vi "SoftwareBreakpoint.vi"(0 "Motion Board ID":T2=1 min=1 max=32 step=1, 1 "Axis or Vector Space":T1=1 items=["Axis 1"=1, "Axis 2"=2, "Axis 3"=3, "Axis 4"=4, "Axis 5"=5, "Axis 6"=6, "Axis 7"=7, "Axis 8"=8, "Vector Space 1"=17, "Vector Space 2"=18, "Vector Space 3"=19, "Vector Space 4"=20], 2 "Start Position":i32=500, 3 "Breakpoint Modulus":i32=500, 4 "error in (no error)":errorcluster) -> (6 "Breakpoints Occured":i32)   [LabVIEW 2022 SP3]
uses:
  <vilib>/Motion/FlexMotion/CustomControls/CustomControls.llb/AxisOrVectorSpace To Control.flx
panel:
  out "BreakPT marks":i32[](array[numeric])
  out "Current Position":i32=2000
  # "Enter a breakpoint Modulus, and the\nBreakpoint Output will occur at 0 and\nincrements of the Modulus Value."
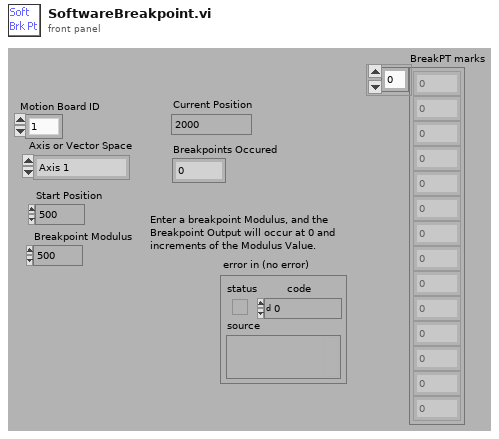
[diagram p1: front panel]
types:
  T1 = typedef "AxisOrVectorSpace To Control.flx" = u16
  T2 = typedef "Board Id" = u8
  T3 = typedef "Resource Out (Enum).flx" = u16
  T4 = typedef "Bd Id Out" = u8
  T5 = cluster{"Run/Stop":bool, "Profile Complete":bool, "Motor Off ":bool, "Following Error":bool, "Limit Switch":bool, "Home Switch":bool, "SW Limit Switch":bool, "Watchdog":bool, "Velocity Threshold":bool, "Position Brkpt":bool, "Home Found":bool, "Index Found":bool, "High Speed Capture":bool, "Reverse Direction":bool, "Blend Complete":bool, "Move Complete":bool}
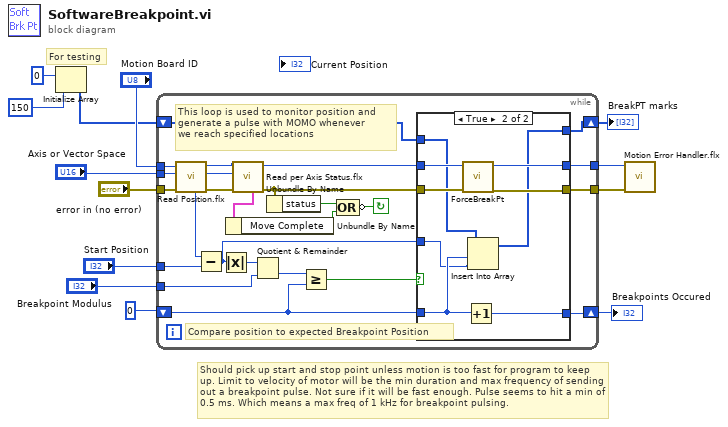
[diagram p0: block diagram]
diagram:
  # "For testing"
  # "Should pick up start and stop point unless motion is too fast for program to keep up. Limit to velocity of motor will be the min duration and max frequency of sending out a breakpoint pulse. Not sure if it will be fast enough. Pulse seems to hit a min of 0.5 ms. Which means a max freq of 1 kHz for breakpoint pulsing."
  n1 = Initialize Array(0, 150) -> (w2:i32[])
  n2 = while {
    shift-left: 0 -> [w18]
    shift-right: [w23] -> w7
    tunnel: "Axis or Vector Space" -> [w26]
    tunnel: "Motion Board ID" -> [w27]
    tunnel: [w28] -> w10
    tunnel: [w29] -> w11
    tunnel: "error in (no error)" -> [w24]
    tunnel: "Breakpoint Modulus" -> [w21]
    tunnel: "Start Position" -> [w20]
    shift-right: [w14] -> w1
    shift-left: w2 -> [w15]
    stop <- w25 continue-if-true
    # "Compare position to expected Breakpoint Position"
    # "This loop is used to monitor position and \ngenerate a pulse with MOMO whenever \nwe reach specified locations"
    n3 = call <vilib>:"Read Position.flx"("error in (no error)"=w24, "Axis"=w26, "Board ID"=w27) -> ("error out"=w33:errorcluster, "Resource Output"=w31:T3, "Bd ID Out"=w32:T4, "Position"=w22:i32)  [unwired: 3 out]
    n4 = Subtract(x=w22, y=w20) -> (x-y=w16:i32)
    n5 = Absolute Value(x=w16) -> (abs(x)=w30:i32)
    n6 = call <vilib>:"Read per Axis Status.flx"("error in (no error)"=w33, "Axis"=w31, "Board ID"=w32) -> ("error out"=w34:errorcluster, "Bd ID Out"=w35:T4, "Per Axis H/W Status"=w38:T5)  [unwired: 4 out]
    n7 = Unbundle By Name(w38) -> ("Move Complete"=w36:bool)
    n8 = Quotient & Remainder(x=w30, y=w21) -> (floor(x/y)=w19:i32)  [unwired: 1 out]
    n9 = Unbundle By Name(w34) -> ("status"=w37:bool)
    n10 = Greater Or Equal?(x=w19, y=w18) -> (x >= y?=w17:bool)
    n11 = Compound Arithmetic op=OR(w37, w36) -> (invert w25:bool)
    n12 = case shown="True" w17 {
      tunnel: w35 -> [w40 w47]
      tunnel: [w40 w50] -> w28
      tunnel: [w42 w49] -> w29
      tunnel: w34 -> [w42 w51]
      tunnel: w18 -> [w41 w45]
      tunnel: [w41 w48] -> w23
      tunnel: w16 -> [_ w44]
      tunnel: w15 -> [w39 w46]
      tunnel: [w39 w43] -> w14
      frame False {
      }
      frame True {
        n13 = call "ForceBreakPt.vi"("error in"=w51, "Bd ID in"=w47) -> ("error out"=w49:errorcluster, "Bd ID Out"=w50:u8)
        n14 = Increment(x=w45) -> (x+1=w48:i32)
        n15 = Insert Into Array(array=w46, index=w45, new element=w44) -> (w43:i32[])
      }
    }
  }
  "Breakpoints Occured" <- w7
  "BreakPT marks" <- w1
  n16 = call <vilib>:"Motion Error Handler.flx"("Board ID"=w10, "error in (no error)"=w11) -> ()  [unwired: 3 in, 11 out]
